vi "stepper driver -- arduino.vi"(6 "Instrument Address":refnum<visa-resource-name>="ASRL3::INSTR", 7 "stepper driver action":T1, 10 "speed IN":dbl, 11 "number":dbl format="%#_13g") -> (1 "stepper motor state OUT":T2, 2 "speed":dbl, 3 "number out":dbl)   [LabVIEW 2018]
uses:
  stepper motor state.ctl
  stepper driver action.ctl
  internal stepper driver state -- arduino.ctl
  <vilib>/regexp/Match Regular Expression.xnode
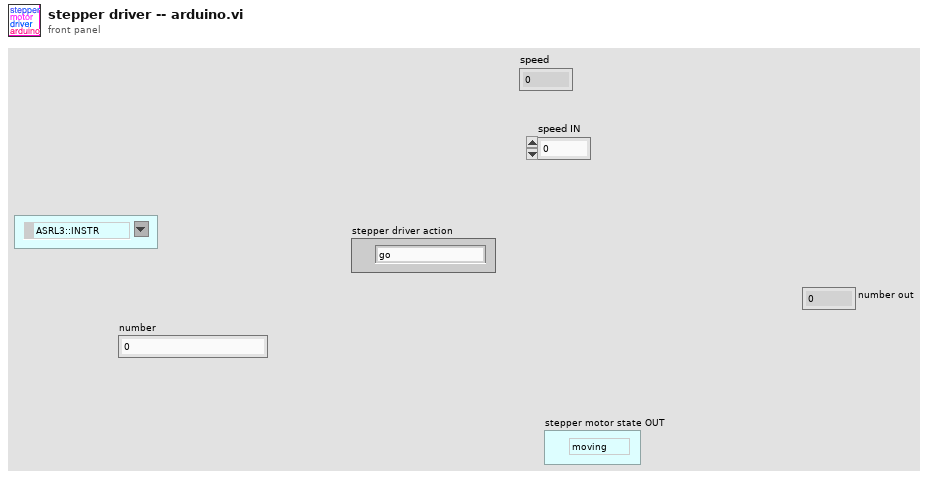
[diagram p1: front panel]
types:
  T1 = typedef "stepper driver action.ctl" = enum16{"go", "void", "stop", "check", "init", "sync", "set", "set speed", "--check status", "--check value", "--handshake"}
  T2 = typedef "stepper motor state.ctl" = enum16{"moving", "stopped"}
  T3 = typedef "internal stepper driver state -- arduino.ctl" = cluster{"VISA address":refnum<visa-resource-name>, "stepper motor state":T2, "Motor Address":u32, "speed":i32, "target position":dbl, "current position":dbl, "ready?":bool, "steps per top deg":dbl}
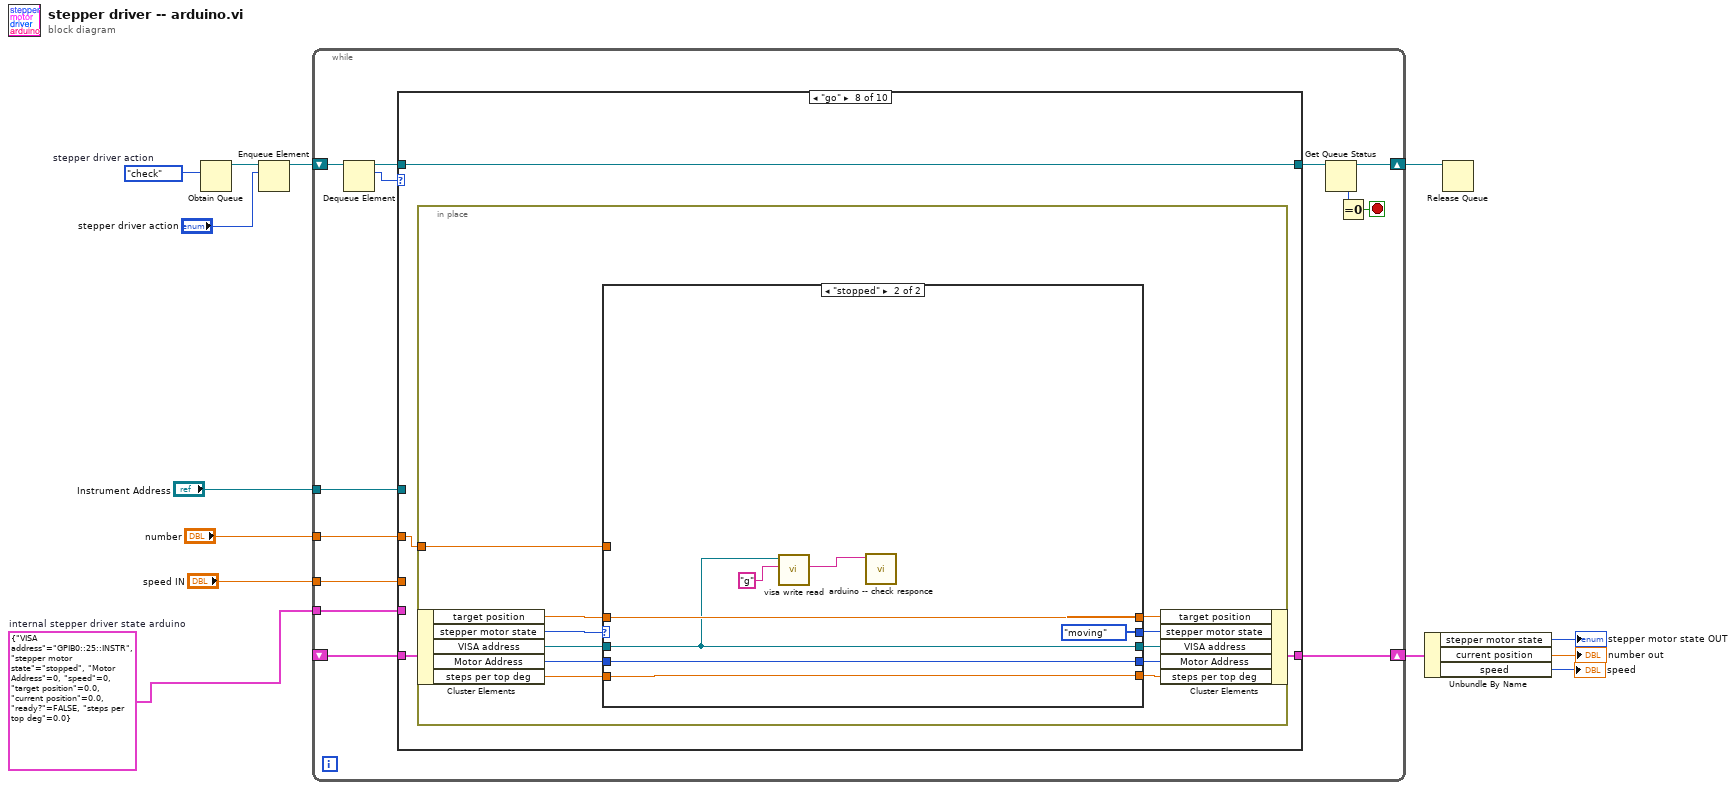
[diagram p0: block diagram]
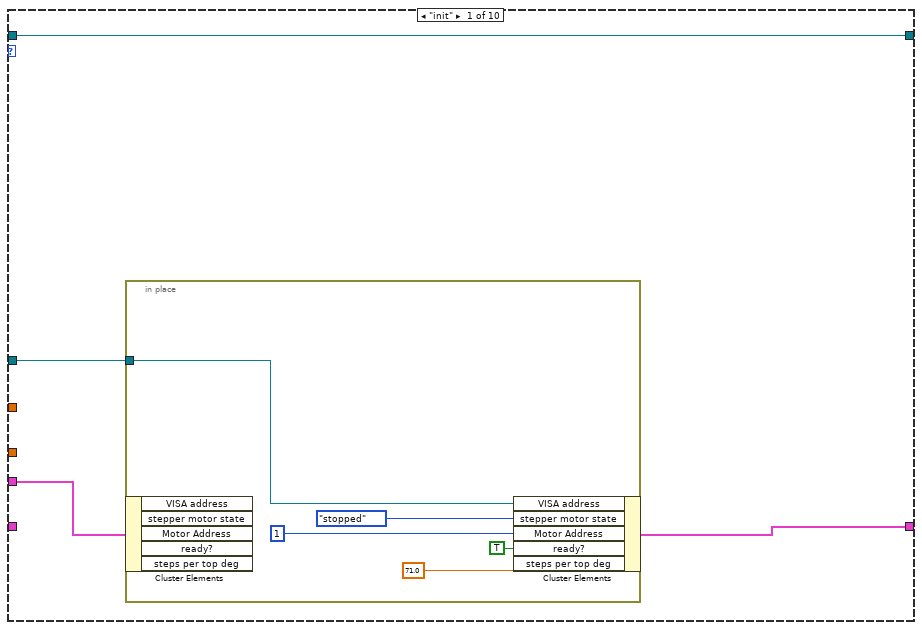
[diagram p2: hidden frame]
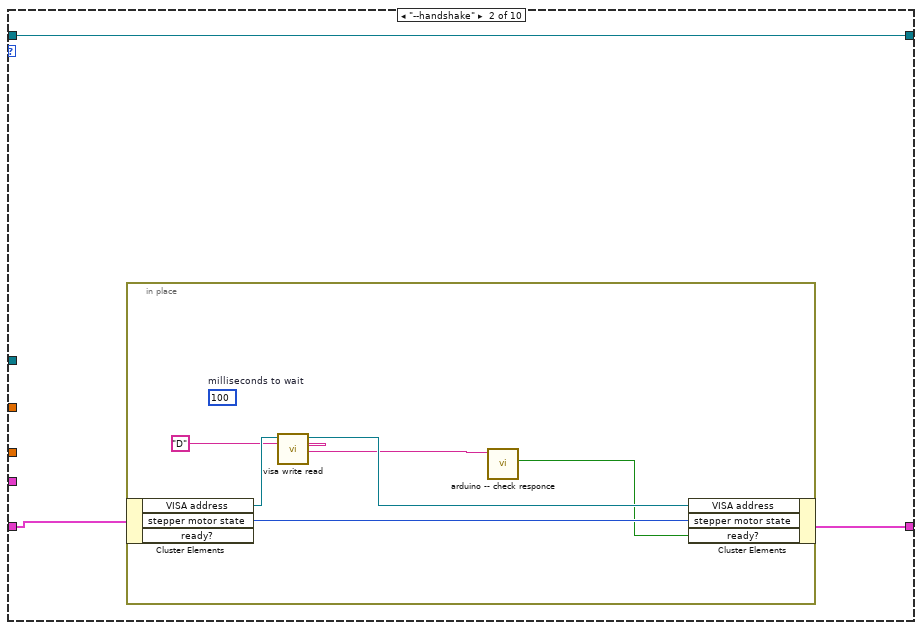
[diagram p3: hidden frame]
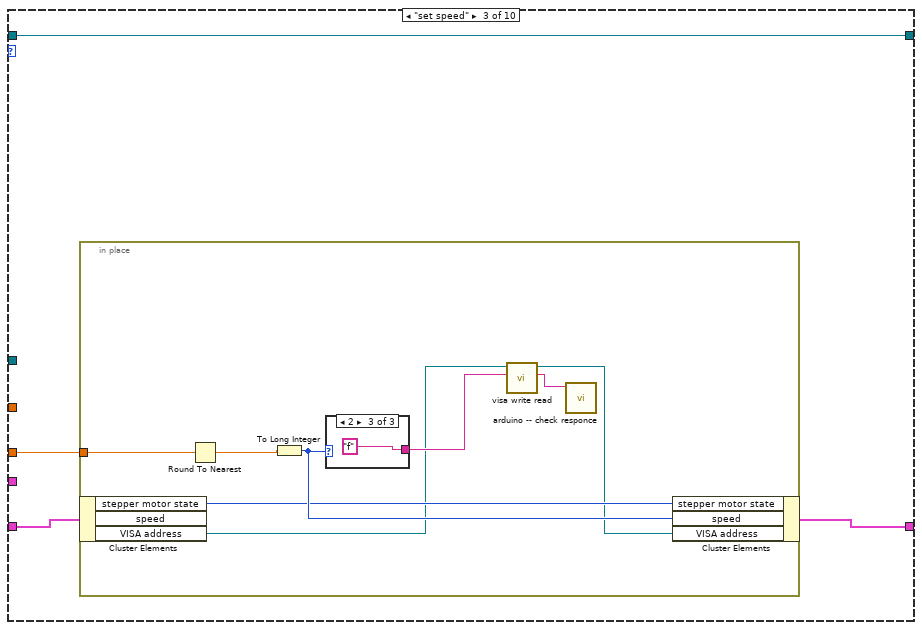
[diagram p4: hidden frame]
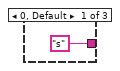
[diagram p5: hidden frame]
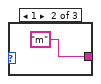
[diagram p6: hidden frame]
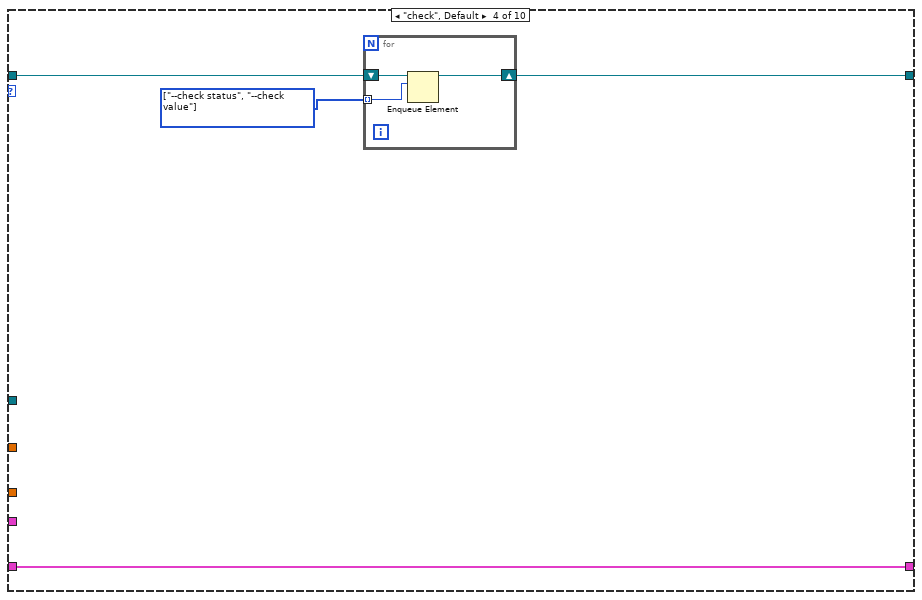
[diagram p7: hidden frame]
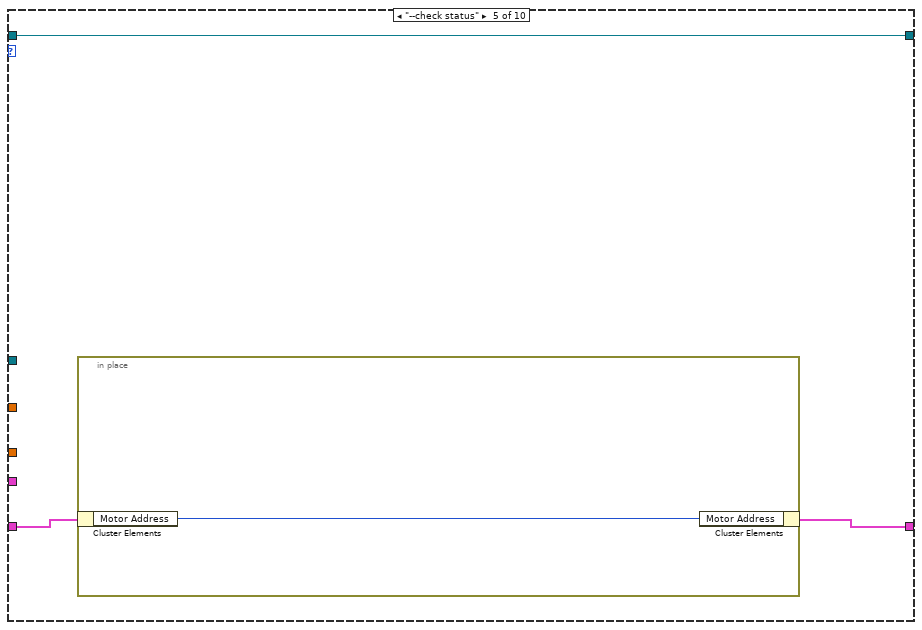
[diagram p8: hidden frame]
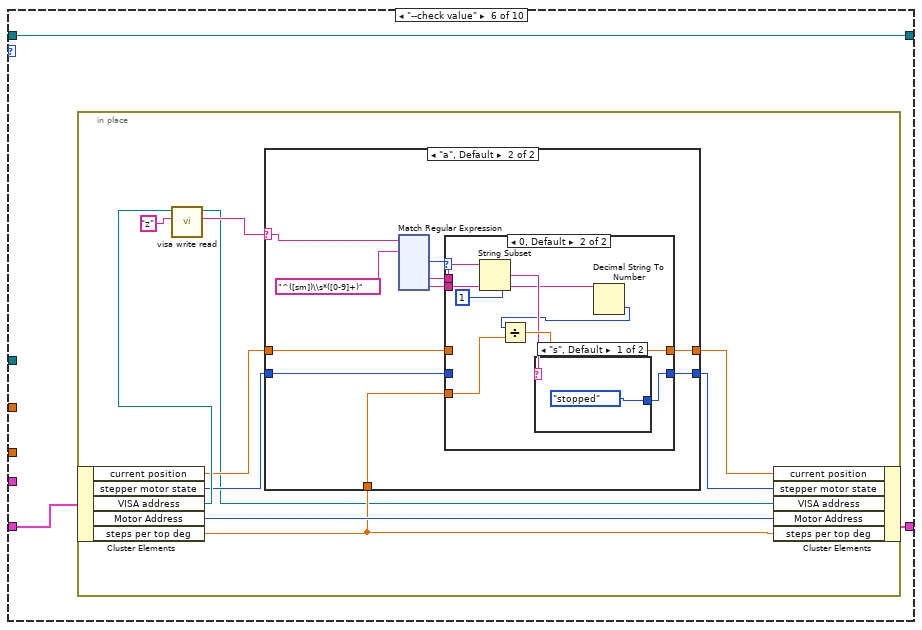
[diagram p9: hidden frame]
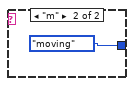
[diagram p12: hidden frame]
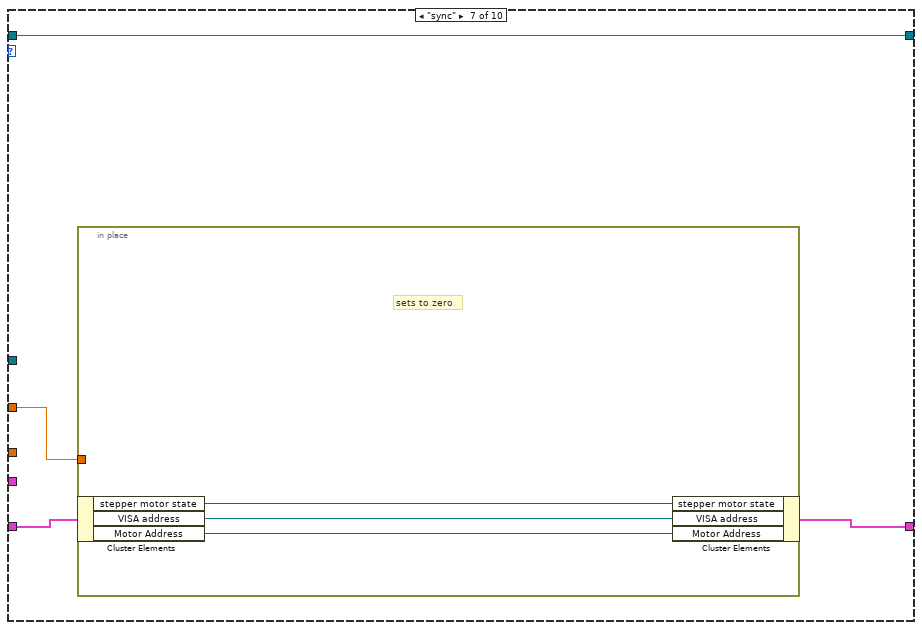
[diagram p13: hidden frame]
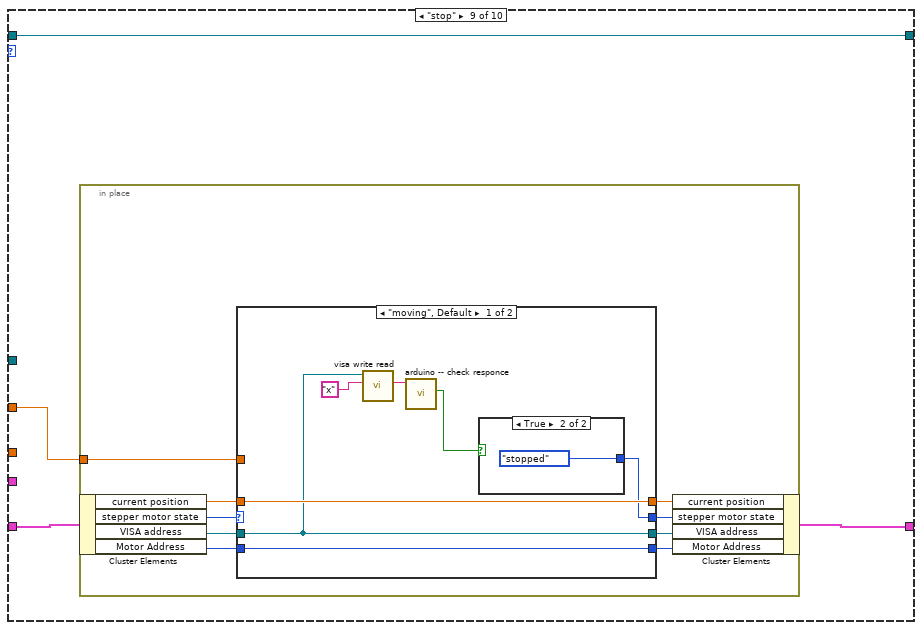
[diagram p15: hidden frame]
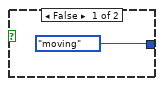
[diagram p16: hidden frame]
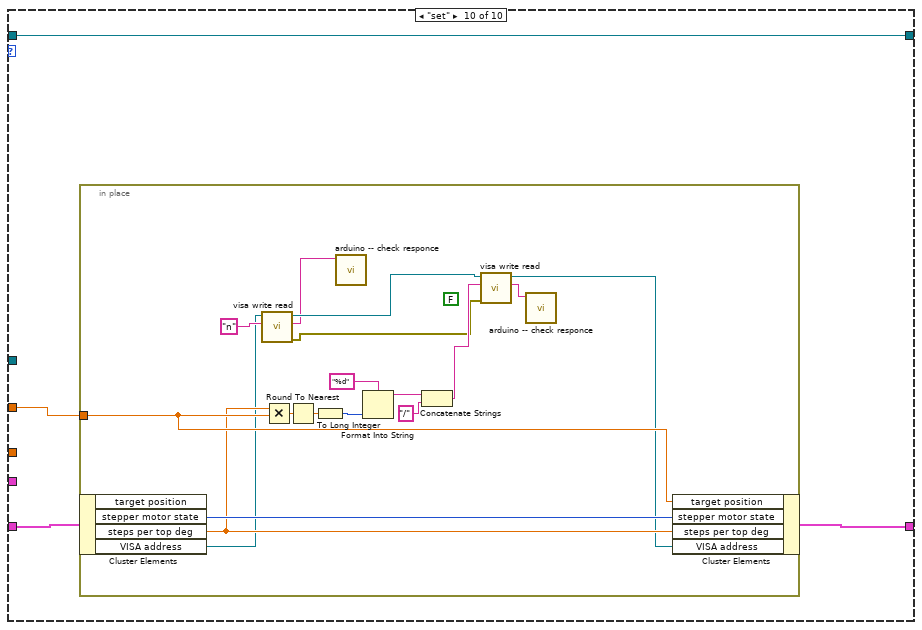
[diagram p18: hidden frame]
diagram:
  w1 = T3 {"VISA address"="GPIB0::25::INSTR", "stepper motor state"=enum."stopped", "Motor Address"=0, "speed"=0, "target position"=0.0, "current position"=0.0, "ready?"=FALSE, "steps per top deg"=0.0}  # internal stepper driver state arduino
  w10 = stepper_driver_action."check"  # stepper driver action
  n1 = Obtain Queue(element data type=w10) -> (queue out=w9:refnum<queue>)  [unwired: 4 in, 2 out]
  n2 = Enqueue Element(queue=w9, element="stepper driver action") -> (queue out=w8:refnum<queue>)  [unwired: 2 in, 2 out]
  n3 = while {
    shift-right: [w26] -> w11
    shift-left: _ -> [w25]
    shift-right: [w18] -> w7
    shift-left: w8 -> [w22]
    tunnel: w1 -> [w24]
    tunnel: "number" -> [w23]
    tunnel: "Instrument Address" -> [w15]
    tunnel: "speed IN" -> [w14]
    stop <- w16 stop-if-true
    n4 = Dequeue Element(queue=w22) -> (queue out=w21:refnum<queue>, element=w20:T1)  [unwired: 2 in, 2 out]
    n5 = case shown="\"go\"" w20 {
      tunnel: [w29 w38 w46 w63 w68 w72 w226 w233 w260 w286] -> w26
      tunnel: w25 -> [_ w36 w47 w63 w69 w73 w227 w234 w261 w287]
      tunnel: [w27 w37 w48 w61 w67 w71 w228 w235 w262 w288] -> w19
      tunnel: w21 -> [w27 w37 w48 w62 w67 w71 w228 w235 w262 w288]
      tunnel: w24 -> [w30 _ _ _ _ _ _ _ _ _]
      tunnel: w23 -> [_ _ _ _ _ _ w225 w232 w259 w285]
      tunnel: w15 -> [w28 _ _ _ _ _ _ _ _ _]
      tunnel: w14 -> [_ _ w45 _ _ _ _ _ _ _]
      frame "init" {
        n6 = in-place {
          in-place-border: w28 -> [w33]
          n7 = in-place-cluster #1(w30) -> ()  [unwired: 5 out]
          n8 = in-place-cluster #1("VISA address"=w33, "stepper motor state"=stepper_motor_state."stopped", "Motor Address"=u32 1, "ready?"=TRUE, "steps per top deg"=71.0) -> (w29:T3)
        }
      }
      frame "--handshake" {
        n9 = in-place {
          (unwired) u32 100  # milliseconds to wait
          n10 = in-place-cluster #2(w36) -> ("VISA address"=w43:refnum<visa-resource-name>, "stepper motor state"=w44:T2)  [unwired: 1 out]
          n11 = call "visa write read.vi"("write buffer"="D", "VISA resource name"=w43) -> ("read buffer"=w40:string, "VISA resource name out"=w42:refnum<visa-resource-name>)  [unwired: 7 in, 1 out]
          n12 = call "arduino -- check responce.vi"("resonse"=w40) -> ("ok?"=w39:bool)  [unwired: 10 in]
          n13 = in-place-cluster #2("VISA address"=w42, "stepper motor state"=w44, "ready?"=w39) -> (w38:T3)
        }
      }
      frame "set speed" {
        n14 = in-place {
          in-place-border: w45 -> [w56]
          n15 = in-place-cluster #3(w47) -> ("stepper motor state"=w51:T2, "VISA address"=w50:refnum<visa-resource-name>)  [unwired: 1 out]
          n16 = Round To Nearest(number=w56) -> (nearest integer value=w55:dbl)
          n17 = To Long Integer(number=w55) -> (32bit integer=w52:i32)
          n18 = case shown="2" w52 {
            tunnel: ["s" "m" "f"] -> w53
            frame 0, Default {
            }
            frame 1 {
            }
            frame 2 {
            }
          }
          n19 = call "visa write read.vi"("write buffer"=w53, "VISA resource name"=w50) -> ("read buffer"=w54:string, "VISA resource name out"=w49:refnum<visa-resource-name>)  [unwired: 7 in, 1 out]
          n20 = call "arduino -- check responce.vi"("resonse"=w54) -> ()  [unwired: 10 in, 1 out]
          n21 = in-place-cluster #3("stepper motor state"=w51, "speed"=w52, "VISA address"=w49) -> (w46:T3)
        }
      }
      frame "check", Default {
        w60 = T1[] [enum."--check status", enum."--check value"] items=["go", "void", "stop", "check", "init", "sync", "set", "set speed", "--check status", "--check value", "--handshake"] ("action list IN")
        n22 = for {
          shift-right: [w65] -> w61
          shift-left: w62 -> [w66]
          tunnel: w60 -> [w64] mode=indexing
          n23 = Enqueue Element(queue=w66, element=w64) -> (queue out=w65:refnum<queue>)  [unwired: 2 in, 2 out]
        }
      }
      frame "--check status" {
        n24 = in-place {
          n25 = in-place-cluster #4(w69) -> ("Motor Address"=w70:u32)
          n26 = in-place-cluster #4("Motor Address"=w70) -> (w68:T3)
        }
      }
      frame "--check value" {
        n27 = in-place {
          n28 = in-place-cluster #5(w73) -> ("current position"=w80:dbl, "stepper motor state"=w77:T2, "VISA address"=w81:refnum<visa-resource-name>, "Motor Address"=w83:u32, "steps per top deg"=w76:dbl)
          n29 = call "visa write read.vi"("write buffer"="z", "VISA resource name"=w81) -> ("read buffer"=w75:string, "VISA resource name out"=w74:refnum<visa-resource-name>)  [unwired: 7 in, 1 out]
          n30 = case shown="\"a\", Default" w75 {
            selector: w75 -> [_ w86]
            tunnel: w80 -> [w85 w91]
            tunnel: w76 -> [_ w95]
            tunnel: [w85 w94] -> w79
            tunnel: [w84 w90] -> w78
            tunnel: w77 -> [w84 w89]
            frame "" {
            }
            frame "a", Default {
              n31 = xnode "Match Regular Expression"("input string"=w86, "regular expression"="^([sm])\\s*([0-9]+)") -> ("offset past match"=w92:i32, "submatch 1"=w88:string, "submatch 2"=w87:string)  [unwired: 4 in, 4 out]
              n32 = case shown="0, Default" w92 {
                tunnel: w95 -> [_ w105]
                tunnel: [w97 w104] -> w94
                tunnel: w91 -> [w97 _]
                tunnel: [w96 w100] -> w90
                tunnel: w89 -> [w96 _]
                tunnel: w88 -> [_ w103]
                tunnel: w87 -> [_ w99]
                frame -1 {
                }
                frame 0, Default {
                  n33 = String Subset(string=w103, length (rest)=1 ("length (rest)")) -> (substring=w101:string)  [unwired: 1 in]
                  n34 = case shown="\"s\", Default" w101 {
                    tunnel: [stepper_motor_state."stopped" ("stepper motor state") stepper_motor_state."moving" ("stepper motor state")] -> w100
                    frame "s", Default {
                    }
                    frame "m" {
                    }
                  }
                  n35 = Decimal String To Number(string=w99) -> (number=w98:i32)  [unwired: 2 in, 1 out]
                  n36 = Divide(x=w98, y=w105) -> (x/y=w104:dbl)
                }
              }
            }
          }
          n37 = in-place-cluster #5("current position"=w79, "stepper motor state"=w78, "VISA address"=w74, "Motor Address"=w83, "steps per top deg"=w76) -> (w72:T3)
        }
      }
      frame "sync" {
        n38 = in-place {
          in-place-border: w225 -> [_]
          # "sets to zero"
          n39 = in-place-cluster #6(w227) -> ("stepper motor state"=w231:T2, "VISA address"=w230:refnum<visa-resource-name>, "Motor Address"=w229:u32)
          n40 = in-place-cluster #6("stepper motor state"=w231, "VISA address"=w230, "Motor Address"=w229) -> (w226:T3)
        }
      }
      frame "go" {
        n41 = in-place {
          in-place-border: w232 -> [w246]
          n42 = in-place-cluster #7(w234) -> ("target position"=w240:dbl, "stepper motor state"=w243:T2, "VISA address"=w245:refnum<visa-resource-name>, "Motor Address"=w244:u32, "steps per top deg"=w237:dbl)
          n43 = case shown="\"stopped\"" w243 {
            selector: w243 -> [w248 _]
            tunnel: w246 -> [_ _]
            tunnel: w245 -> [w251 w252]
            tunnel: w244 -> [w250 w257]
            tunnel: [w251 w252] -> w242
            tunnel: [w250 w257] -> w241
            tunnel: w240 -> [w249 w258]
            tunnel: [w248 stepper_motor_state."moving" ("stepper motor state")] -> w239
            tunnel: [w249 w258] -> w238
            tunnel: w237 -> [w247 w256]
            tunnel: [w247 w256] -> w236
            frame "moving", Default {
            }
            frame "stopped" {
              n44 = call "visa write read.vi"("write buffer"="g", "VISA resource name"=w252) -> ("read buffer"=w254:string)  [unwired: 7 in, 2 out]
              n45 = call "arduino -- check responce.vi"("resonse"=w254) -> ()  [unwired: 10 in, 1 out]
            }
          }
          n46 = in-place-cluster #7("target position"=w238, "stepper motor state"=w239, "VISA address"=w242, "Motor Address"=w241, "steps per top deg"=w236) -> (w233:T3)
        }
      }
      frame "stop" {
        n47 = in-place {
          in-place-border: w259 -> [w271]
          n48 = in-place-cluster #8(w261) -> ("current position"=w263:dbl, "stepper motor state"=w268:T2, "VISA address"=w270:refnum<visa-resource-name>, "Motor Address"=w269:u32)
          n49 = case shown="\"moving\", Default" w268 {
            selector: w268 -> [_ w282]
            tunnel: w271 -> [_ _]
            tunnel: w270 -> [w274 w284]
            tunnel: w269 -> [w278 w283]
            tunnel: [w274 w284] -> w267
            tunnel: [w278 w283] -> w266
            tunnel: [w272 w282] -> w265
            tunnel: [w277 w281] -> w264
            tunnel: w263 -> [w277 w281]
            frame "moving", Default {
              n50 = call "visa write read.vi"("write buffer"="x", "VISA resource name"=w274) -> ("read buffer"=w275:string)  [unwired: 7 in, 2 out]
              n51 = call "arduino -- check responce.vi"("resonse"=w275) -> ("ok?"=w273:bool)  [unwired: 10 in]
              n52 = case shown="True" w273 {
                tunnel: [stepper_motor_state."moving" ("stepper motor state") stepper_motor_state."stopped" ("stepper motor state")] -> w272
                frame False {
                }
                frame True {
                }
              }
            }
            frame "stopped" {
            }
          }
          n53 = in-place-cluster #8("current position"=w264, "stepper motor state"=w265, "VISA address"=w267, "Motor Address"=w266) -> (w260:T3)
        }
      }
      frame "set" {
        n54 = in-place {
          in-place-border: w285 -> [w297]
          (unwired) FALSE
          n55 = in-place-cluster #9(w287) -> ("stepper motor state"=w298:T2, "steps per top deg"=w296:dbl, "VISA address"=w292:refnum<visa-resource-name>)  [unwired: 1 out]
          n56 = call "visa write read.vi"("write buffer"="n", "VISA resource name"=w292) -> ("error out"=w289:errorcluster, "read buffer"=w290:string, "VISA resource name out"=w291:refnum<visa-resource-name>)  [unwired: 7 in]
          n57 = Multiply(x=w296, y=w297) -> (x*y=w303:dbl)
          n58 = Round To Nearest(number=w303) -> (nearest integer value=w301:dbl)
          n59 = To Long Integer(number=w301) -> (32bit integer=w302:i32)
          n60 = call "arduino -- check responce.vi"("resonse"=w290) -> ()  [unwired: 10 in, 1 out]
          n61 = Format Into String(format string="%d", w302) -> (resulting string=w300:string)  [unwired: 2 in, 1 out]
          n62 = Concatenate Strings(w300, "/" ("string")) -> (w294:string)
          n63 = call "visa write read.vi"("error in (no error)"=w289, "write buffer"=w294, "VISA resource name"=w291) -> ("read buffer"=w305:string, "VISA resource name out"=w295:refnum<visa-resource-name>)  [unwired: 6 in, 1 out]
          n64 = call "arduino -- check responce.vi"("resonse"=w305) -> ()  [unwired: 10 in, 1 out]
          n65 = in-place-cluster #9("target position"=w297, "stepper motor state"=w298, "steps per top deg"=w296, "VISA address"=w295) -> (w286:T3)
        }
      }
    }
    n66 = Get Queue Status(queue=w19) -> (queue out=w18:refnum<queue>, # elements in queue=w17:i32)  [unwired: 2 in, 6 out]
    n67 = Equal To 0?(x=w17) -> (x = 0?=w16:bool)
  }
  n68 = Unbundle By Name(w11) -> ("stepper motor state"=→"stepper motor state OUT":T2, "current position"=→"number out":dbl, "speed"=→"speed":i32)
  n69 = Release Queue(queue=w7) -> ()  [unwired: 2 in, 3 out]
